vi "WLAN - niVST - OPPO - RFSG - Generate Script.vi"(0 "Initial Delay (ms)":dbl, 5 "Number of Packets":i32=50 min=1 max=1000, 7 "WaveformNamePostfix":string) -> (6 "resulting script":string)   [LabVIEW 2012]
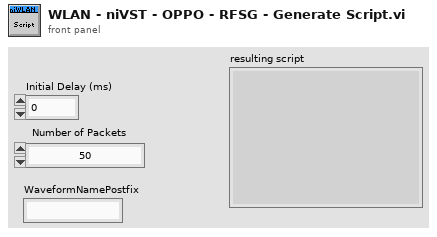
[diagram p1: front panel]
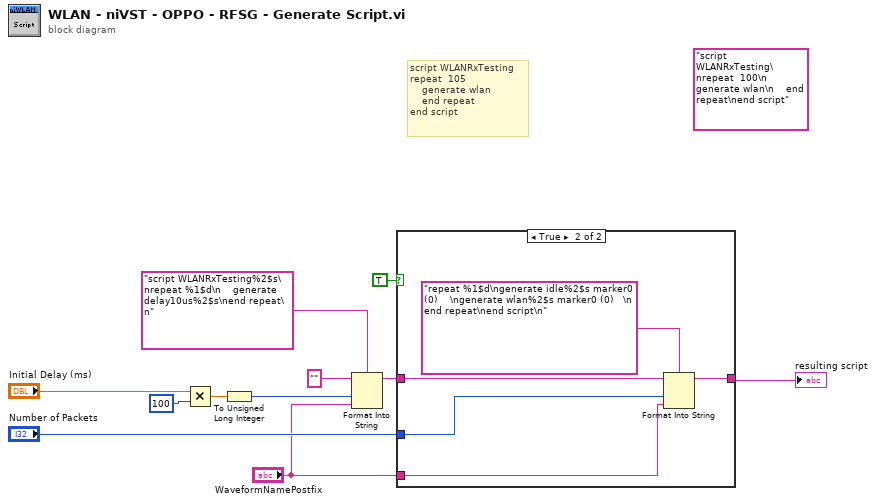
[diagram p0: block diagram]
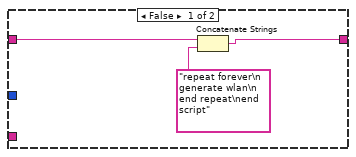
[diagram p2: hidden frame]
diagram:
  (unwired) "script WLANRxTesting\nrepeat  100\n    generate wlan\n    end repeat\nend script" ("Script")
  # "script WLANRxTesting\nrepeat  105\n    generate wlan\n    end repeat\nend script"
  n1 = Multiply(x="Initial Delay (ms)", y=u32 100) -> (x*y=w5:dbl)
  n2 = To Unsigned Long Integer(number=w5) -> (unsigned 32bit integer=w4:u32)
  n3 = Format Into String(format string="script WLANRxTesting%2$s\nrepeat %1$d\n    generate delay10us%2$s\nend repeat\n" ("Script"), initial string="", w4, "WaveformNamePostfix") -> (resulting string=w8:string)  [unwired: 1 in, 1 out]
  n4 = case shown="True" TRUE {
    tunnel: w8 -> [w14 w19]
    tunnel: "Number of Packets" -> [_ w18]
    tunnel: [w12 w16] -> w2
    tunnel: "WaveformNamePostfix" -> [_ w15]
    frame False {
      n5 = Concatenate Strings(w14, "repeat forever\n    generate wlan\n    end repeat\nend script" ("Script")) -> (w12:string)
    }
    frame True {
      n6 = Format Into String(format string="repeat %1$d\ngenerate idle%2$s marker0 (0)    \ngenerate wlan%2$s marker0 (0)   \n    end repeat\nend script\n" ("Script"), initial string=w19, w18, w15) -> (resulting string=w16:string)  [unwired: 1 in, 1 out]
    }
  }
  "resulting script" <- w2
